vi "DAQNavi String To Enum.vi"(2 "enumString":string, 3 "enumTypeName":string) -> (1 "enumValue":i32)   [LabVIEW 2020]
uses:
  DAQNavi_LV.dll
panel:
  out "return type":i32
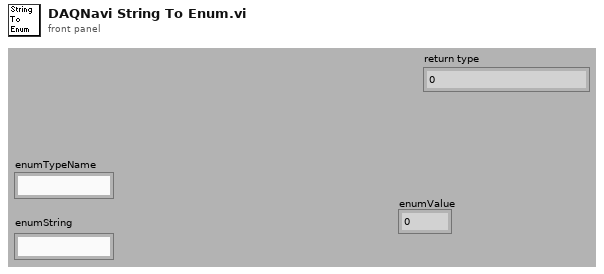
[diagram p1: front panel]
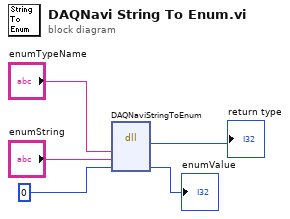
[diagram p0: block diagram]
diagram:
  n1 = dll-call lib="DAQNavi_LV.dll" fn="DAQNaviStringToEnum"("enumTypeName"="enumTypeName", "enumString"="enumString", "enumValue"=0) -> ("return type"=→"return type":i32, "enumValue"=→"enumValue":i32)  [unwired: 5 in, 2 out]
